vi "verifyMotorController.vi"(7 "error in (no error)":errorcluster, 9 "interface object in":refnum<k20>, 10 "MotorControllerClass in":refnum<class "MotorControllerClass.lvclass">) -> (0 "error out":errorcluster, 1 "isCorrectController":bool, 2 "interface object out":refnum<k20>, 3 "MotorControllerClass out":refnum<class "MotorControllerClass.lvclass">)   [LabVIEW 2018, in "MotorControllerClass.lvclass"]
uses:
  BMS/MotorControllerClass.lvclass
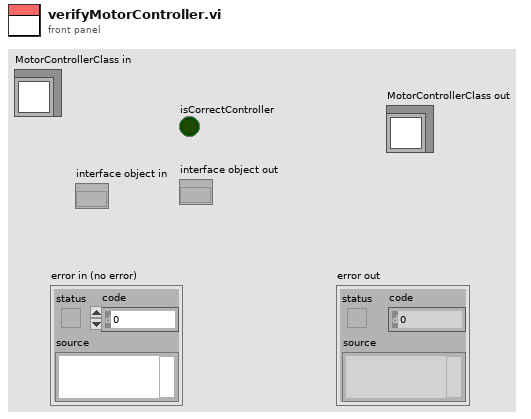
[diagram p1: front panel]
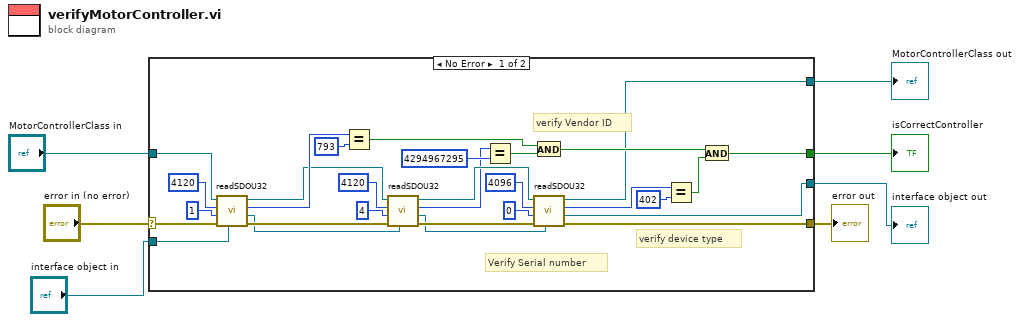
[diagram p0: block diagram]
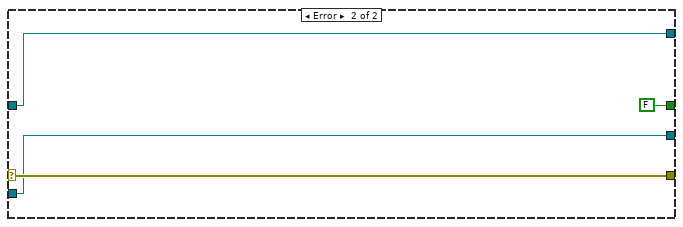
[diagram p2: hidden frame]
diagram:
  n1 = case shown="No Error" "error in (no error)" {
    selector: "error in (no error)" -> [w27 w40]
    tunnel: [w14 w40] -> w6
    tunnel: [w13 w37] -> w1
    tunnel: [w11 w38] -> w5
    tunnel: "interface object in" -> [w28 w38]
    tunnel: [w31 FALSE] -> w3
    tunnel: "MotorControllerClass in" -> [w24 w37]
    frame No Error {
      # "verify device type"
      # "verify Vendor ID"
      # "Verify Serial number"
      n2 = call "readSDOU32.vi"("interface object in"=w28, "error in (no error)"=w27, "subIndex"=u8 1, "objectIndex"=u16 4120, "MotorControllerClass in"=w24) -> ("error out"=w19:errorcluster, "interface object out"=w8:refnum<k20>, "output"=w23:u32, "MotorControllerClass out"=w20:refnum<class "MotorControllerClass.lvclass">)  [unwired: 3 in]
      n3 = Equal?(x=w23, y=u32 793) -> (x = y?=w35:bool)
      n4 = call "readSDOU32.vi"("interface object in"=w8, "error in (no error)"=w19, "subIndex"=u8 4, "objectIndex"=u16 4120, "MotorControllerClass in"=w20) -> ("error out"=w15:errorcluster, "interface object out"=w10:refnum<k20>, "output"=w9:u32, "MotorControllerClass out"=w18:refnum<class "MotorControllerClass.lvclass">)  [unwired: 3 in]
      n5 = Equal?(x=w9, y=u32 4294967295) -> (x = y?=w34:bool)
      n6 = And(x=w35, y=w34) -> (x .and. y?=w32:bool)
      n7 = call "readSDOU32.vi"("interface object in"=w10, "error in (no error)"=w15, "subIndex"=u8 0, "objectIndex"=u16 4096, "MotorControllerClass in"=w18) -> ("error out"=w14:errorcluster, "interface object out"=w11:refnum<k20>, "output"=w12:u32, "MotorControllerClass out"=w13:refnum<class "MotorControllerClass.lvclass">)  [unwired: 3 in]
      n8 = Equal?(x=w12, y=u32 402) -> (x = y?=w29:bool)
      n9 = And(x=w32, y=w29) -> (x .and. y?=w31:bool)
    }
    frame Error {
    }
  }
  "error out" <- w6
  "interface object out" <- w5
  "isCorrectController" <- w3
  "MotorControllerClass out" <- w1
